vi "Write Version from ini File.vi"(8 "error in":errorcluster, 9 "Entry":string, 10 "index of element":i32, 11 "Page Refnum":refnum<vi>) -> (0 "error out":errorcluster, 3 "Page Refnum":refnum<vi>)   [LabVIEW 2014]
doc: "It writes the version number obtained from the ini file (for Push function)."
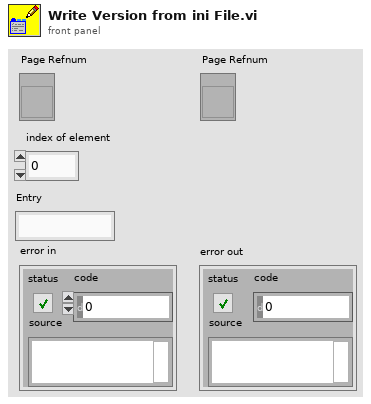
[diagram p1: front panel]
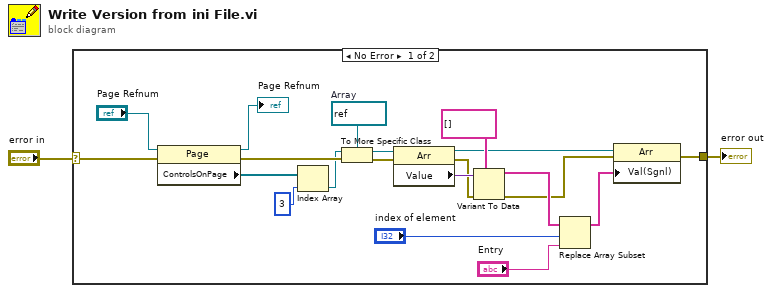
[diagram p0: block diagram]
diagram:
  n1 = case shown="No Error" "error in" {
    selector: "error in" -> [w14 w23]
    tunnel: [w3 w23] -> w2
    frame No Error {
      w17 = refnum<vi> refnum  # Array
      n2 = property class="Page"(reference="Page Refnum", error in=w14) -> (reference out=→"Page Refnum":refnum<vi>, error out=w19:errorcluster, "ControlsOnPage"=w21:refnum<vi>[])
      n3 = Index Array(array=w21, index=3) -> (element=w16:refnum<vi>)
      n4 = To More Specific Class(target class=w17, reference=w16, error in=w19) -> (specific class reference=w15:refnum<vi>, error out=w18:errorcluster)
      n5 = property class="Arr"(reference=w15, error in=w18) -> (reference out=w6:refnum<vi>, error out=w10:errorcluster, "Value"=w12:variant)
      n6 = Variant To Data(error in=w10, type=string[] [], Variant=w12) -> (data=w9:string[], error out=w5:errorcluster)
      n7 = Replace Array Subset(array=w9, new element="Entry", index="index of element") -> (w4:string[])
      n8 = property class="Arr"(reference=w6, error in=w5, "Val(Sgnl)"=w4) -> (error out=w3:errorcluster)  [unwired: 1 out]
    }
    frame Error {
    }
  }
  "error out" <- w2
